vi "HIOKI PW3390 Configuration Motor Analysis.vi"() -> ()   [LabVIEW 2009]
doc: "Sets the configuration and outputs the measurement data about the motor analysis."
uses:
  <instrlib>/PW3390/Configure/Motor/_CH B/HIOKI PW3390 Conf CH B Pulse.vi
  <instrlib>/PW3390/Configure/Motor/_CH A/HIOKI PW3390 Conf CH A DC.vi
  <instrlib>/PW3390/Common/_Initialize/HIOKI PW3390 Initialize LAN.vi
  <instrlib>/PW3390/Common/_Initialize/HIOKI PW3390 Initialize RS-232C.vi
panel:
  in  "Item":T1(array[cluster])=[{"Item"=enum."CH A", "Ch(0:Ch1)"=enum."1"}, {"Item"=enum."CH B", "Ch(0:Ch1)"=enum."1"}, {"Item"=enum."Pm", "Ch(0:Ch1)"=enum."1"}, {"Item"=enum."Slip", "Ch(0:Ch1)"=enum."1"}]
  out "error out":errorcluster
  in  "Communication Interface":enum16{"LAN", "RS-232C"}(ring)
  in  "COM Port":refnum<visa-resource-name>="COM1"
  in  "baud rate (38400bps)":u32=38400
  in  "IP Address":string="192.168.1.1"
  in  "CH Z input (0: OFF)":enum16{"OFF", "ON", "BPHASE"}(ring)
  in  "Motorpoles (4)":i32=4 min=2 max=98 step=2
  in  "Number (2)":i32=2 min=1 max=60000
  in  "Max Frequency (3: 5kHz)":enum16{"100Hz", "500Hz", "1kHz", "5kHz"}(ring)=enum."5kHz"
  in  "Unit (2: rpm)":enum16{"V", "Hz", "rpm"}(ring)=enum."rpm"
  in  "Slip (0: f1)":enum16{"f1", "f2", "f3", "f4"}(ring)
  in  "LPF (0: OFF)":enum16{"OFF", "ON"}(ring)
  in  "Sync source (9: DC50m)":T2(ring)=enum."DC50ms"
  in  "Unit (3: Nm)":enum16{"V", "Hz", "mNm", "Nm", "kNm"}(ring)=enum."Nm"
  in  "Scaling (1.00)":dbl=1.0 min=0.01 max=9999.99 format="%.2f"
  in  "Range (1: 5V)":enum16{"1", "5", "10"}(ring)=enum."5"
  out "Data out":dbl[](array[numeric])
  in  "Stop":bool
  # "Note:\n CH configuration of the Item after CH A is unnecessary."
  # "Note:\n Please set configuration before starting the program.\nChanging configuration during running the program is invalid."
  # "CH B input"
  # "Motor Common input"
  # "CH A input"
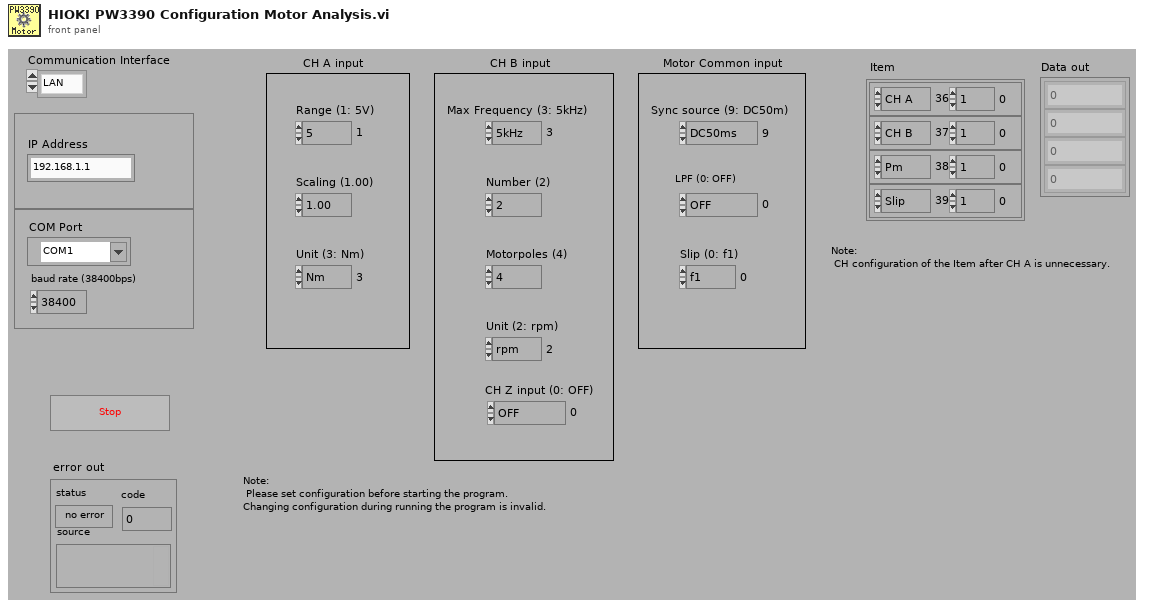
[diagram p1: front panel]
types:
  T1 = cluster{"Item":enum16{"Urms", "Umn", "Uac", "Udc", "Ufnd", "Upk+", "Upk-", "Uthd", "Urf", "Uunb", "Irms", "Imn", "Iac", "Idc", "Ifnd", "Ipk+", "Ipk-", "Ithd", "Irf", "Iunb", "P", "S", "Q", "PF", "DEG U", "DEG I", "DEG P", "f", "EFFI", "LOSS", "IH+", "IH-", "IH", "WP+", "WP-", "WP", "CH A", "CH B", "Pm", "Slip", "Laptime", "Laptime(ms)"}, "Ch(0:Ch1)":enum16{"1", "2", "3", "4", "12", "34", "123"}}[]
  T2 = enum16{"U1", "U2", "U3", "U4", "I1", "I2", "I3", "I4", "Ext", "DC50ms", "DC100ms"}
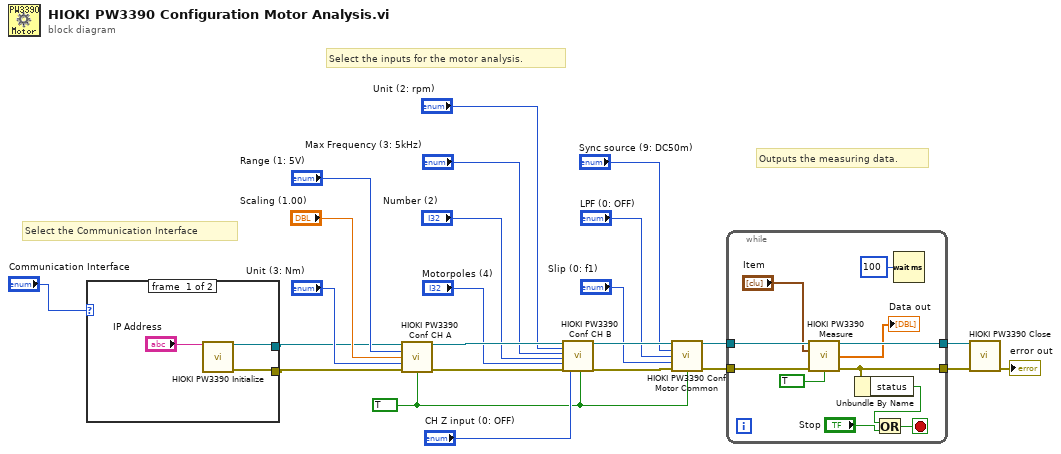
[diagram p0: block diagram]
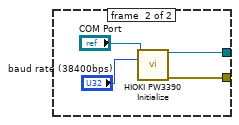
[diagram p2: hidden frame]
diagram:
  w1 = TRUE ("Error Out (F: Off)")
  # "Select the Communication Interface"
  # "Outputs the measuring data."
  # "Select the inputs for the motor analysis."
  n1 = case shown="\"LAN\", デフォルト" "Communication Interface" {
    tunnel: [w26 w31] -> w3
    tunnel: [w25 w30] -> w4
    frame #0 {
      n2 = call-poly <instrlib>:"HIOKI PW3390 Initialize.vi"("IP Address"="IP Address") -> ("VISA Resource out"=w26:refnum<visa-resource-name>, "error out"=w25:errorcluster)  [unwired: 12 in, 1 out]
    }
    frame #1 {
      n3 = call-poly <instrlib>:"HIOKI PW3390 Initialize.vi"("COM Port"="COM Port", "baud rate (38400bps)"="baud rate (38400bps)") -> ("VISA Resource out"=w31:refnum<visa-resource-name>, "error out"=w30:errorcluster)  [unwired: 11 in, 1 out]
    }
  }
  n4 = call-poly <instrlib>:"HIOKI PW3390 Conf CH A.vi"("VISA Resource"=w3, "Range (1: 5V)"="Range (1: 5V)", "Scaling (1.00)"="Scaling (1.00)", "Unit (3: Nm)"="Unit (3: Nm)", "error in (no error)"=w4, "Error Out (F: Off)"=w1) -> ("VISA Resource out"=w22:refnum<visa-resource-name>, "error out"=w21:errorcluster)  [unwired: 4 in, 4 out]
  n5 = call-poly <instrlib>:"HIOKI PW3390 Conf CH B.vi"("VISA Resource"=w22, "Unit (2: rpm)"="Unit (2: rpm)", "Max Frequency (3: 5kHz)"="Max Frequency (3: 5kHz)", "Number (2)"="Number (2)", "Motorpoles (4)"="Motorpoles (4)", "error in (no error)"=w21, "CH Z input (0: OFF)"="CH Z input (0: OFF)", "Error Out (F: Off)"=w1) -> ("VISA Resource out"=w20:refnum<visa-resource-name>, "error out"=w19:errorcluster)  [unwired: 4 in, 6 out]
  n6 = call <instrlib>:"HIOKI PW3390 Conf Motor Common.vi"("VISA Resource"=w20, "Sync Source (9: DC50m)"="Sync source (9: DC50m)", "LPF (0: OFF)"="LPF (0: OFF)", "Slip (0: f1)"="Slip (0: f1)", "error in (no error)"=w19, "Error Out (F: Off)"=w1) -> ("VISA Resource out"=w24:refnum<visa-resource-name>, "error out"=w23:errorcluster)  [unwired: 5 in, 3 out]
  n7 = while {
    tunnel: w24 -> [w42]
    tunnel: w23 -> [w41]
    tunnel: [w40] -> w18
    tunnel: [w37] -> w17
    stop <- w36 stop-if-true
    n8 = call <instrlib>:"HIOKI PW3390 Measure.vi"("VISA Resource"=w42, "Item"="Item", "error in (no error)"=w41, "Error Out (F: Off)"=TRUE) -> ("VISA Resource out"=w40:refnum<visa-resource-name>, "Data out"=→"Data out":dbl[], "error out"=w37:errorcluster)  [unwired: 6 in, 3 out]
    n9 = Unbundle By Name(w37) -> ("status"=w34:bool)
    n10 = Or(x=w34, y="Stop") -> (x .or. y?=w36:bool)
    n11 = Wait (ms)(milliseconds to wait=u32 100) -> ()  [unwired: 1 out]
  }
  n12 = call <instrlib>:"HIOKI PW3390 Close.vi"("VISA Resource"=w18, "error in (no error)"=w17) -> ("error out"=→"error out":errorcluster)  [unwired: 13 in]
